vi "Main_flow_full_mqtt_with_power_calculation.vi"() -> ()   [LabVIEW 2022 SP3]
uses:
  D:/UOM/EE2044 - Electrical Measurements and Instrumentation/Project/Measurment Project/Quaxo_MQTT_LabVIEW-master/Controls/Connection_Return_Codes.ctl
  D:/UOM/EE2044 - Electrical Measurements and Instrumentation/Project/Measurment Project/Quaxo_MQTT_LabVIEW-master/Controls/QoS.ctl
  D:/UOM/EE2044 - Electrical Measurements and Instrumentation/Project/Measurment Project/Quaxo_MQTT_LabVIEW-master/Controls/Retain_Flag.ctl
  D:/UOM/EE2044 - Electrical Measurements and Instrumentation/Project/Measurment Project/Quaxo_MQTT_LabVIEW-master/Controls/DUP_Flag.ctl
  D:/UOM/EE2044 - Electrical Measurements and Instrumentation/Project/Measurment Project/Quaxo_MQTT_LabVIEW-master/Controls/Connect_Flags.ctl
  D:/UOM/EE2044 - Electrical Measurements and Instrumentation/Project/Measurment Project/Quaxo_MQTT_LabVIEW-master/Controls/User_Info.ctl
  <vilib>/DAQmx/write.llb/DAQmx Write (Digital Bool 1Line 1Point).vi
  <vilib>/DAQmx/read.llb/DAQmx Read (Digital Bool 1Line 1Point).vi
  <vilib>/DAQmx/create/channels.llb/DAQmx Create Channel (DO-Digital Output).vi
  <vilib>/DAQmx/create/channels.llb/DAQmx Create Channel (DI-Digital Input).vi
  <vilib>/DAQmx/miscellaneous.llb/DAQmx Fill In Error Info.vi
  <vilib>/DAQmx/create/channels.llb/DAQmx Create Channel (AI-Voltage-Basic).vi
  <vilib>/DAQmx/read.llb/DAQmx Read (Analog 1D DBL NChan 1Samp).vi
  D:/UOM/EE2044 - Electrical Measurements and Instrumentation/Project/Measurment Project/Quaxo_MQTT_LabVIEW-master/MQTT_Functions.lvlib
panel:
  out "Current":dbl caption="Current (A)"
  out "Energy":dbl caption="Energy( Whr)"
  in  "clock stop":bool
  out "Time":string
  out "Servo Angle":dbl(knob) scale=0.0..150.0
  in  "stop (F)":bool
  out "PWM Wave":dynamicdata(graph) caption="Square"
  in  "Frequency":dbl=50.0
  in  "Offset":dbl=2.5
  in  "Amplitude":dbl=2.5
  in  "MQTT Broker":cluster{"address (IP)":string, "port":u16}={"address (IP)"="broker.mqttdashboard.com", "port"=1883}
  out "Counter":dbl
  out "OUT COUNT":dbl
  out "IN COUNT":dbl
  in  "Mode":dbl
  in  "Relay 2":tag
  in  "Relay 1":tag
  in  "UP DOWN 2":tag
  in  "UP DOWN 1":tag
  in  "Buzzer":tag
  in  "Door IR 1 & 2 & LDR & Current":tag
  out "LDR Value":dbl(knob) scale=0.0..10.0
  in  "Trigger Period(sec)":dbl
  out "?":bool
  out "?":bool
  out "?":bool
  in  "mqtt stop":bool
  in  "Publish Meta":cluster{"QoS":T1, "Retain":T2, "DUP":T3}
  out "Connection Status":T4=enum."Connection refused: not authorized"
  in  "Client ID":string="NodeE-12345"
  out "main loop executed":dbl
  out "Current Time":dbl
  in  "stop":bool
  # "Channel Configure"
  # "MQTT Configure"
  # "MQTT publish interval\nset channels\nset check mode trigger period"
  # "Dev1/ai4:7"
  # "Dev1/port0/line2"
  # "Dev1/port0/line0"
  # "Dev1/port0/line1"
  # "Dev1/port0/line3"
  # "Dev1/port0/line4"
  # "Dev1/port0/line4"
  # "Servo Motor Controller"
  # "Counter Status"
  # "Light Mode"
  # "Low"
  # "Medium"
  # "High"
  # "This Indicate the status of light mode in the room"
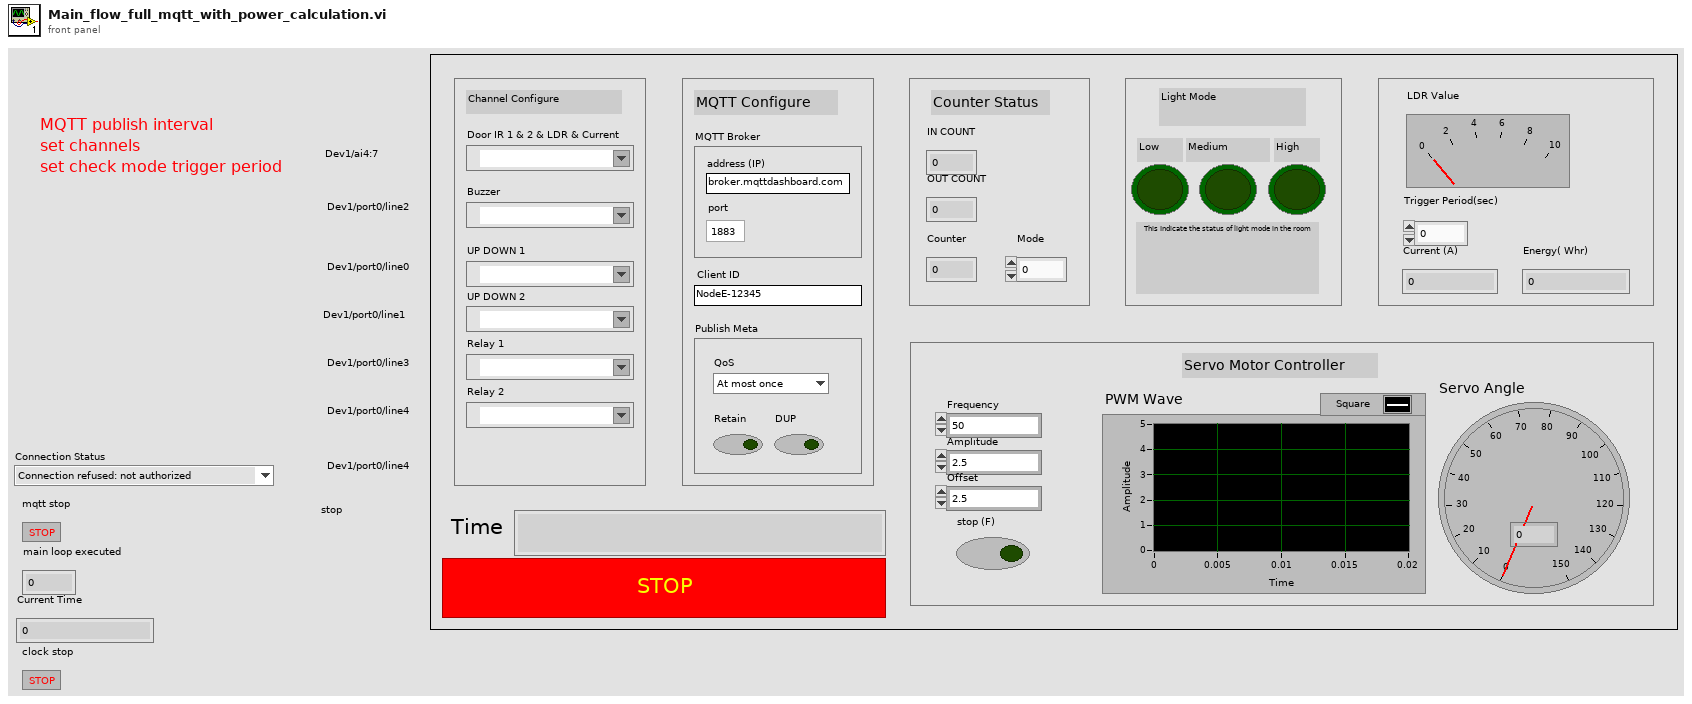
[diagram p1: front panel]
types:
  T1 = typedef "MQTT_Functions.lvlib/QoS.ctl" = enum8{"At most once", "At least once", "Exactly once", "Reserved"}
  T2 = typedef "MQTT_Functions.lvlib/Retain_Flag.ctl" = bool
  T3 = typedef "MQTT_Functions.lvlib/DUP_Flag.ctl" = bool
  T4 = typedef "MQTT_Functions.lvlib/Connection_Return_Codes.ctl" = enum16{"Connection accepted", "Connection refused: unacceptable protocol version", "Connection refused: identifier rejected", "Connection refused: Server unavailable", "Connection refused: bad user name or password", "Connection refused: not authorized"}
  T5 = typedef "MQTT_Functions.lvlib/User_Info.ctl" = cluster{"User Name":string, "Password":string}
  T6 = typedef "MQTT_Functions.lvlib/Connect_Flags.ctl" = cluster{"user name":bool, "password":bool, "will retain":bool, "will flag":bool, "clean session":bool, "reserved":bool, "will QoS":T1}
  T7 = cluster{"QoS":T1, "DUP":T3, "Retain":T2, "Keep Alive (sec)":u16}
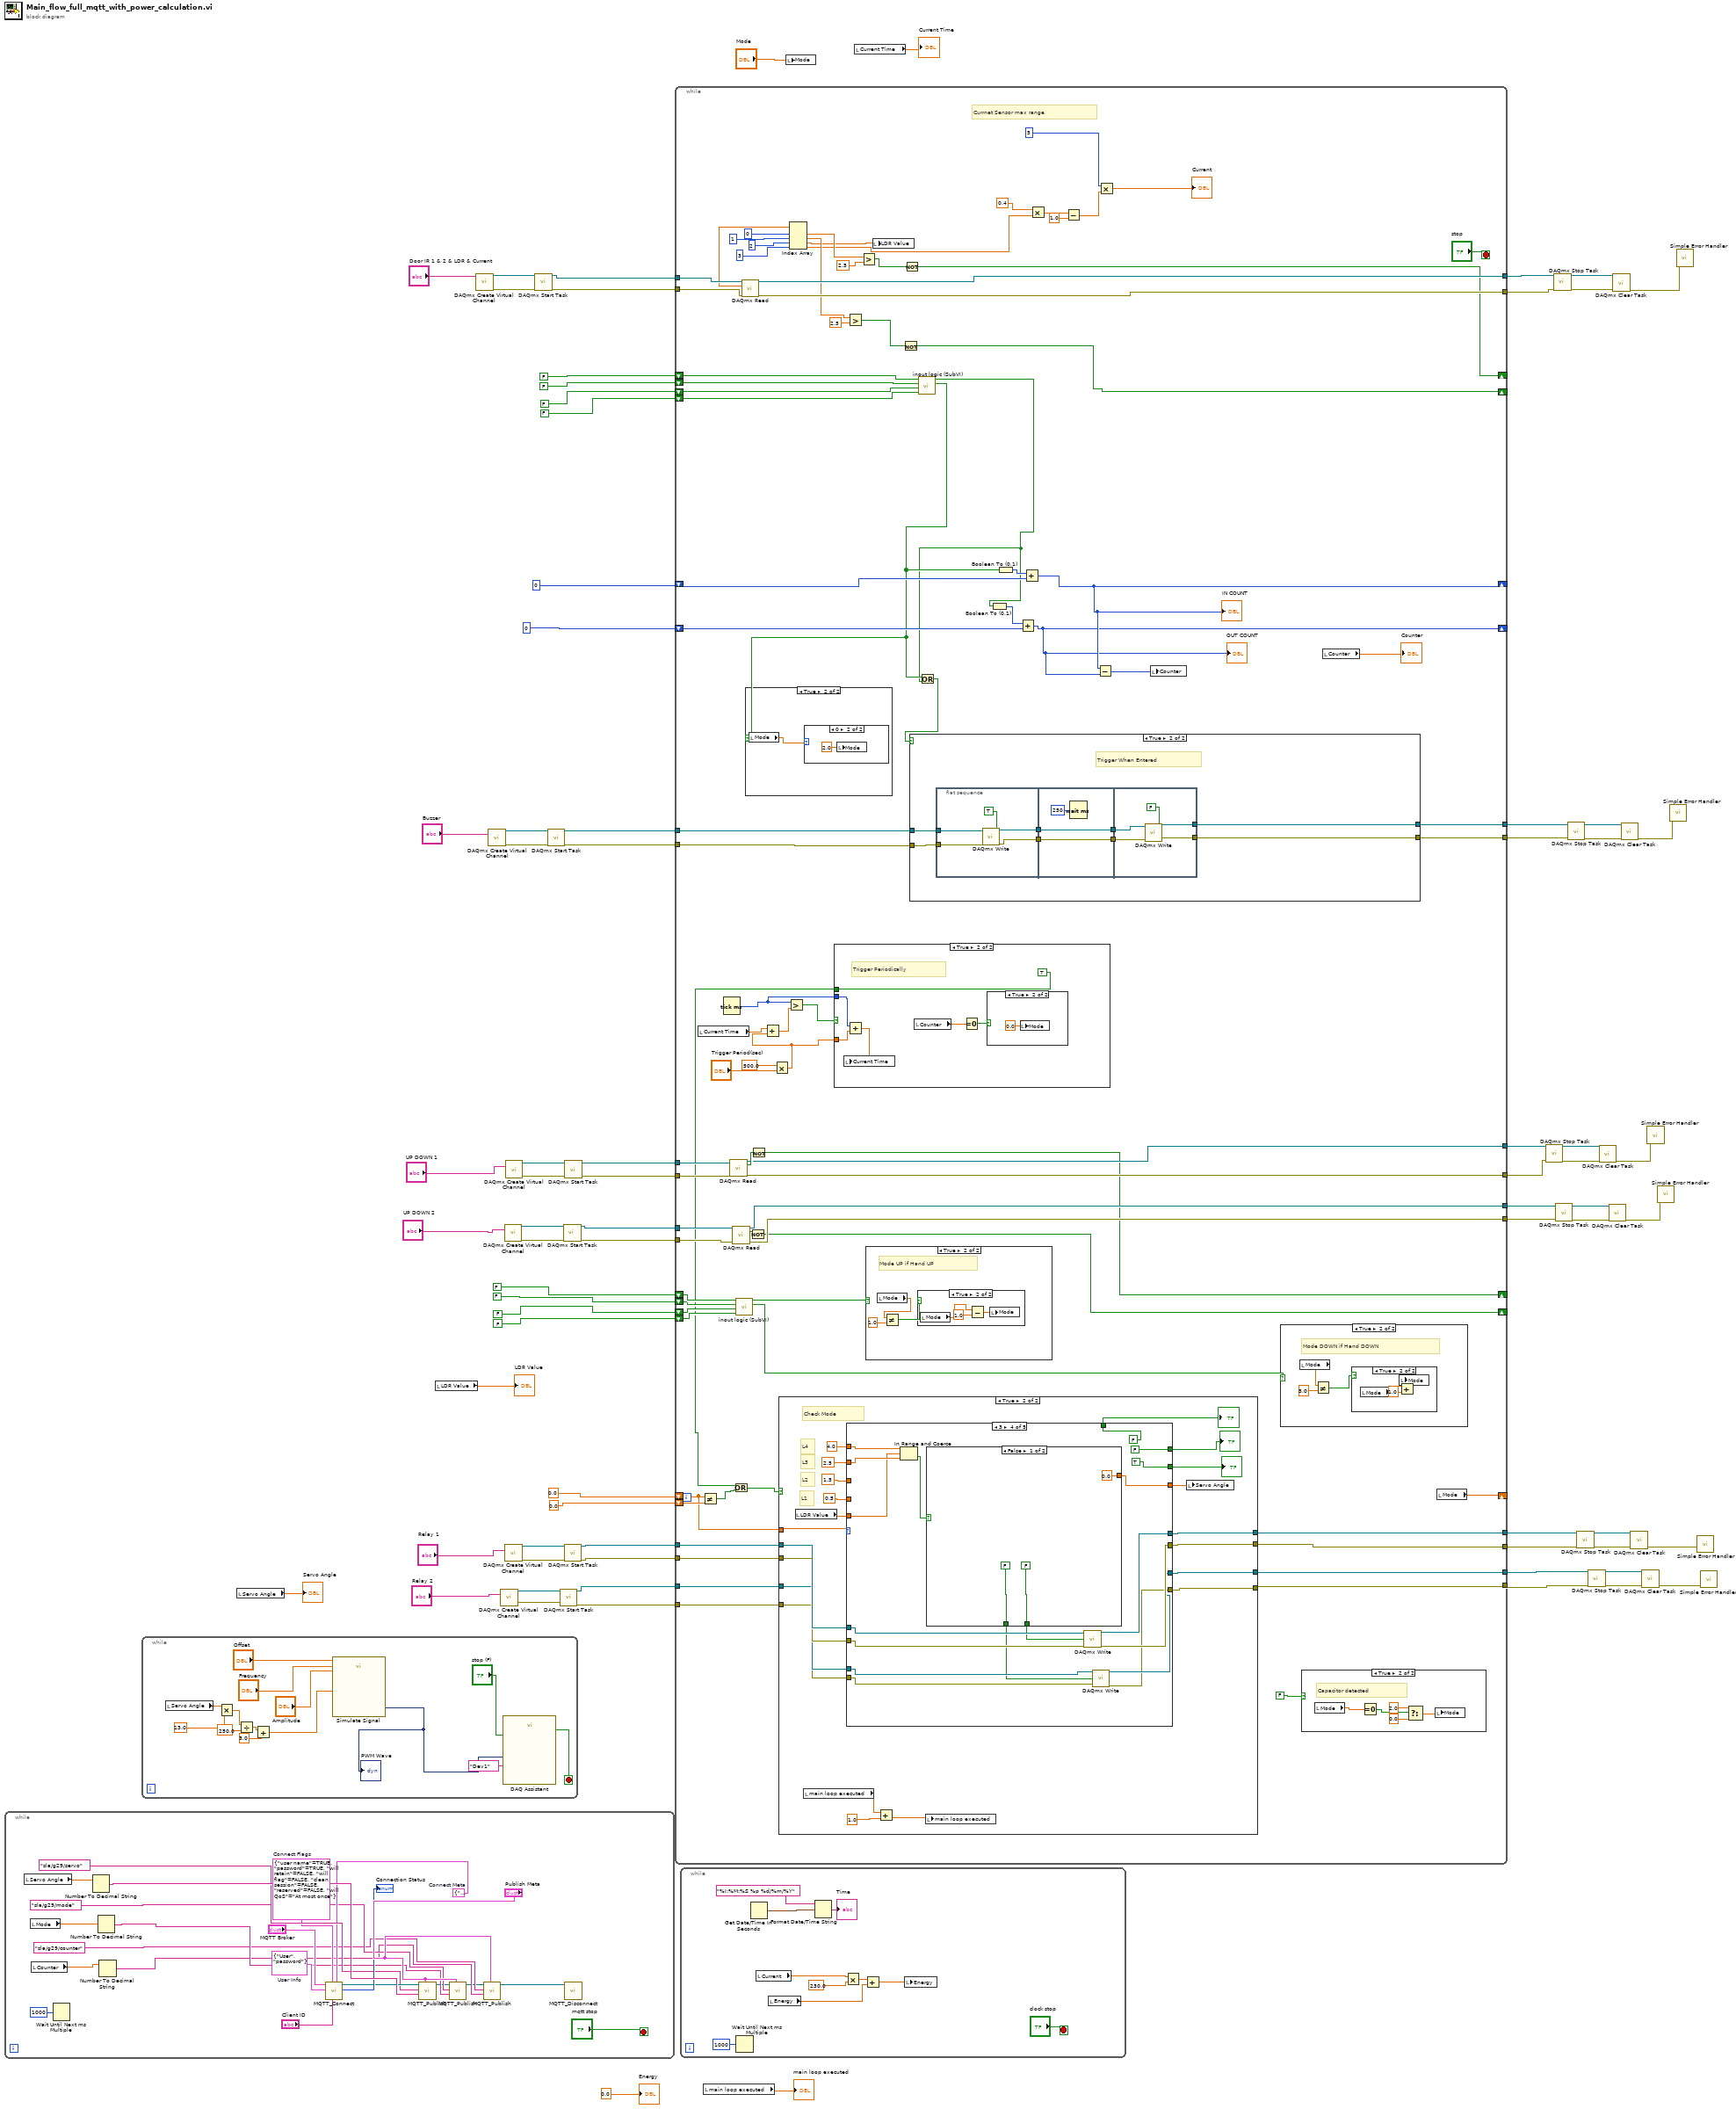
[diagram p0: block diagram]
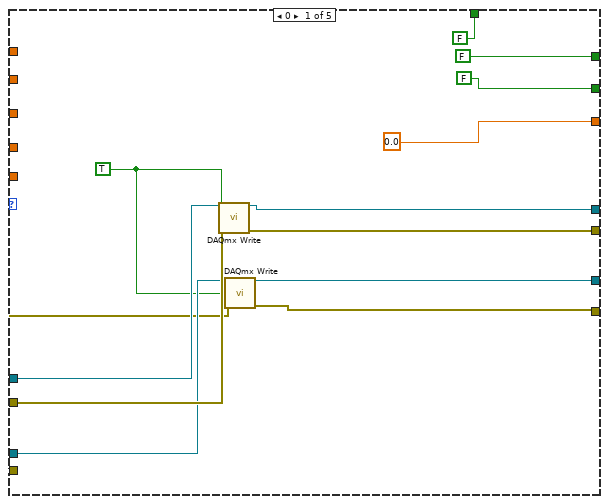
[diagram p5: hidden frame]
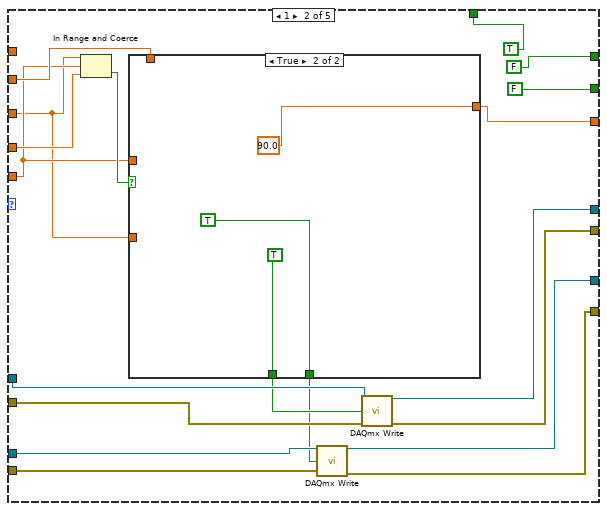
[diagram p6: hidden frame]
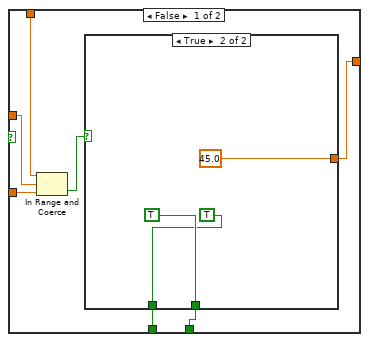
[diagram p7: hidden frame]
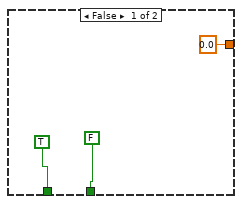
[diagram p8: hidden frame]
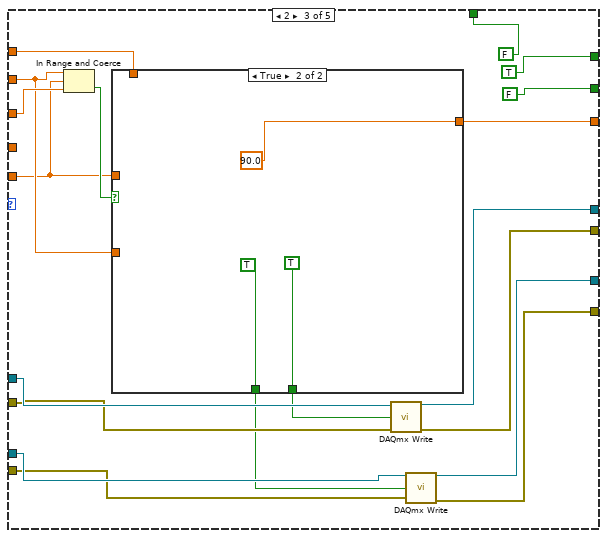
[diagram p9: hidden frame]
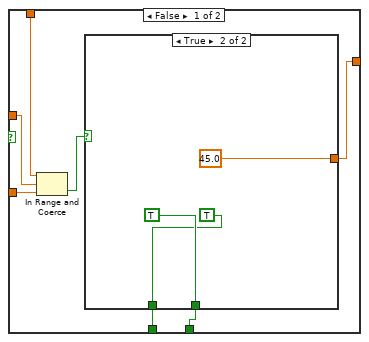
[diagram p10: hidden frame]
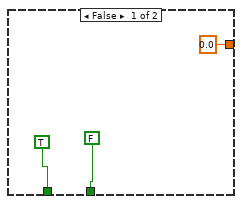
[diagram p11: hidden frame]
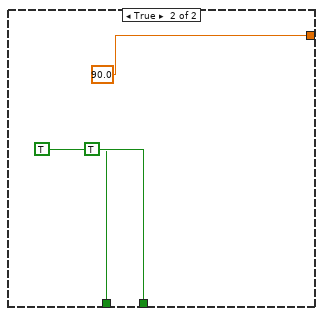
[diagram p12: hidden frame]
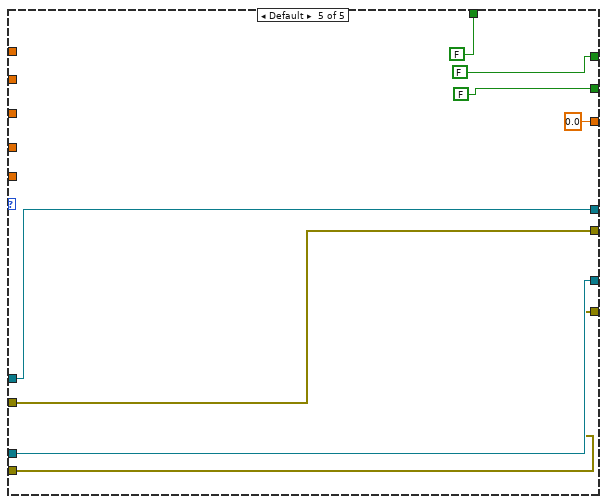
[diagram p13: hidden frame]
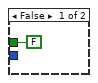
[diagram p18: hidden frame]
diagram:
  n1 = while {
    stop <- "mqtt stop" stop-if-true
    w86 = T5 {"User Name"="User", "Password"="password"}  # User Info
    w87 = T6 {"user name"=TRUE, "password"=TRUE, "will retain"=FALSE, "will flag"=FALSE, "clean session"=FALSE, "reserved"=FALSE, "will QoS"=enum."At most once"}  # Connect Flags
    w88 = T7 {"QoS"=enum."At most once", "DUP"=FALSE, "Retain"=FALSE, "Keep Alive (sec)"=60}  # Connect Meta
    n2 = local read "Servo Angle"() -> (w97:dbl)
    n3 = local read "Mode"() -> (w99:dbl)
    n4 = local read "Counter"() -> (w98:dbl)
    n5 = Wait Until Next ms Multiple(millisecond multiple=u32 1000) -> ()  [unwired: 1 out]
    n6 = Number To Decimal String(number=w97) -> (decimal integer string=w96:string)  [unwired: 1 in]
    n7 = Number To Decimal String(number=w99) -> (decimal integer string=w85:string)  [unwired: 1 in]
    n8 = Number To Decimal String(number=w98) -> (decimal integer string=w83:string)  [unwired: 1 in]
    n9 = call "MQTT_Connect.vi"("Connect Meta"=w88, "Client ID"="Client ID", "Connect Flags"=w87, "User Info"=w86, "MQTT Broker"="MQTT Broker") -> ("Connection Status"=→"Connection Status":T4, "connection ID out"=w93:refnum<k5>)  [unwired: 4 in, 1 out]
    n10 = call "MQTT_Publish.vi"("Publish Meta"="Publish Meta", "Message to be published"=w96, "Topic"="sla/g29/servo", "connection ID"=w93) -> ("connection ID out"=w80:refnum<k5>)  [unwired: 6 in, 1 out]
    n11 = call "MQTT_Publish.vi"("Publish Meta"="Publish Meta", "Message to be published"=w85, "Topic"="sla/g29/mode", "connection ID"=w80) -> ("connection ID out"=w79:refnum<k5>)  [unwired: 6 in, 1 out]
    n12 = call "MQTT_Publish.vi"("Publish Meta"="Publish Meta", "Message to be published"=w83, "Topic"="sla/g29/counter", "connection ID"=w79) -> ("connection ID out"=w91:refnum<k5>)  [unwired: 6 in, 1 out]
    n13 = call "MQTT_Disconnect.vi"("connection ID"=w91) -> ()  [unwired: 10 in, 1 out]
  }
  n14 = while {
    stop <- w113 stop-if-true
    n15 = local read "Servo Angle"() -> (w101:dbl)
    n16 = Multiply(x=w101, y=13.0) -> (x*y=w107:dbl)
    n17 = Divide(x=w107, y=250.0) -> (x/y=w106:dbl)
    n18 = Add(x=w106, y=3.0) -> (x+y=w102:dbl)
    n19 = call "Simulate Signal"("Offset"="Offset", "Duty Cycle (%)"=w102, "Frequency"="Frequency", "Amplitude"="Amplitude") -> ("Square"=w109:dynamicdata)  [unwired: 10 in, 1 out]
    "PWM Wave" <- w109
    n20 = call "DAQ Assistant"("data"=w109, "stop (F)"="stop (F)", "device name"=tag "Dev1") -> ("stopped"=w113:bool)  [unwired: 14 in, 2 out]
  }
  n21 = local read "Servo Angle"() -> (→"Servo Angle":dbl)
  n22 = local read "LDR Value"() -> (→"LDR Value":dbl)
  n23 = call-poly <vilib>:"DAQmx Create Virtual Channel.vi"("physical channels"="Door IR 1 & 2 & LDR & Current") -> ("task out"=w74:refnum<k21>, "error out"=w71:errorcluster)  [unwired: 13 in]
  n24 = call-poly <vilib>:"DAQmx Create Virtual Channel.vi"("lines"="Buzzer") -> ("task out"=w59:refnum<k21>, "error out"=w57:errorcluster)  [unwired: 13 in]
  n25 = call-poly <vilib>:"DAQmx Create Virtual Channel.vi"("lines"="Relay 2") -> ("task out"=w20:refnum<k21>, "error out"=w19:errorcluster)  [unwired: 13 in]
  n26 = call-poly <vilib>:"DAQmx Create Virtual Channel.vi"("lines"="UP DOWN 2") -> ("task out"=w48:refnum<k21>, "error out"=w46:errorcluster)  [unwired: 13 in]
  n27 = call-poly <vilib>:"DAQmx Create Virtual Channel.vi"("lines"="Relay 1") -> ("task out"=w23:refnum<k21>, "error out"=w22:errorcluster)  [unwired: 13 in]
  n28 = call-poly <vilib>:"DAQmx Create Virtual Channel.vi"("lines"="UP DOWN 1") -> ("task out"=w49:refnum<k21>, "error out"=w47:errorcluster)  [unwired: 13 in]
  n29 = call <vilib>:"DAQmx Start Task.vi"("task/channels in"=w74, "error in"=w71) -> ("task out"=w72:refnum<k21>, "error out"=w70:errorcluster)  [unwired: 12 in]
  n30 = call <vilib>:"DAQmx Start Task.vi"("task/channels in"=w59, "error in"=w57) -> ("task out"=w56:refnum<k21>, "error out"=w55:errorcluster)  [unwired: 12 in]
  n31 = call <vilib>:"DAQmx Start Task.vi"("task/channels in"=w20, "error in"=w19) -> ("task out"=w15:refnum<k21>, "error out"=w14:errorcluster)  [unwired: 12 in]
  n32 = call <vilib>:"DAQmx Start Task.vi"("task/channels in"=w48, "error in"=w46) -> ("task out"=w41:refnum<k21>, "error out"=w40:errorcluster)  [unwired: 12 in]
  n33 = call <vilib>:"DAQmx Start Task.vi"("task/channels in"=w23, "error in"=w22) -> ("task out"=w17:refnum<k21>, "error out"=w16:errorcluster)  [unwired: 12 in]
  n34 = call <vilib>:"DAQmx Start Task.vi"("task/channels in"=w49, "error in"=w47) -> ("task out"=w43:refnum<k21>, "error out"=w42:errorcluster)  [unwired: 12 in]
  n35 = while {
    shift-right: [w191] -> _
    shift-left: 0.0 ("Mode") -> [w189]
    shift-left: 0.0 ("Mode") -> [w190]
    tunnel: w72 -> [w186]
    tunnel: w70 -> [w185]
    tunnel: [w184] -> w69
    tunnel: [w183] -> w68
    shift-right: [w174] -> _
    shift-left: FALSE -> [w182]
    shift-left: FALSE -> [w181]
    shift-right: [w177] -> _
    shift-left: FALSE -> [w180]
    shift-left: FALSE -> [w151]
    shift-right: [w176] -> _
    shift-left: 0 -> [w179]
    shift-right: [w175] -> _
    shift-left: 0 -> [w178]
    tunnel: w56 -> [w171]
    tunnel: w55 -> [w170]
    tunnel: [w169] -> w51
    tunnel: [w168] -> w50
    shift-right: [w157] -> _
    shift-left: FALSE -> [w155]
    shift-right: [w156] -> _
    shift-left: FALSE -> [w153]
    shift-left: FALSE -> [w154]
    shift-left: FALSE -> [w152]
    tunnel: w43 -> [w165]
    tunnel: w42 -> [w164]
    tunnel: w41 -> [w163]
    tunnel: w40 -> [w162]
    tunnel: [w161] -> w33
    tunnel: [w160] -> w32
    tunnel: [w159] -> w31
    tunnel: [w158] -> w30
    tunnel: w17 -> [w133]
    tunnel: w16 -> [w132]
    tunnel: w15 -> [w131]
    tunnel: w14 -> [w130]
    tunnel: [w129] -> w7
    tunnel: [w128] -> w6
    tunnel: [w127] -> w5
    tunnel: [w126] -> w4
    stop <- "stop" stop-if-true
    # "Currnet Sensor max range"
    n36 = local read "Current Time"() -> (w198:dbl)
    n37 = Not Equal?(x=w189, y=w190) -> (x != y?=w125:bool)
    n38 = Tick Count (ms)() -> (millisecond timer value=w196:u32)
    n39 = call-poly <vilib>:"DAQmx Read.vi"("task/channels in"=w165, "error in"=w164) -> ("task out"=w161:refnum<k21>, "data"=w167:bool, "error out"=w160:errorcluster)  [unwired: 11 in]
    n40 = call-poly <vilib>:"DAQmx Read.vi"("task/channels in"=w163, "error in"=w162) -> ("task out"=w159:refnum<k21>, "data"=w166:bool, "error out"=w158:errorcluster)  [unwired: 11 in]
    n41 = call "inout logic (SubVI).vi"("Sensor 2 (T-2)"=w152, "Sensor 2 (T-1)"=w153, "Sensor 1 (T-2)"=w154, "Sensor 1 (T-1)"=w155) -> ("IN"=w150:bool, "OUT"=w149:bool)  [unwired: 6 in]
    n42 = call-poly <vilib>:"DAQmx Read.vi"("task/channels in"=w186, "error in"=w185) -> ("task out"=w184:refnum<k21>, "data"=w143:dbl[], "error out"=w183:errorcluster)  [unwired: 11 in]
    n43 = Not(x=w166) -> (.not. x?=w156:bool)
    n44 = Not(x=w167) -> (.not. x?=w157:bool)
    n45 = Multiply(x=500.0, y="Trigger Period(sec)") -> (x*y=w192:dbl)
    n46 = Add(x=w198, y=w192) -> (x+y=w195:dbl)
    n47 = Greater?(x=w196, y=w195) -> (0:w197:bool)
    n48 = Index Array(array=w143, index #1=0 ("index"), index #2=1 ("index"), index #3=2 ("index"), index #4=3 ("index")) -> (element #1=w142:dbl, element #2=w139:dbl, element #3=w134:dbl, element #4=w115:dbl)
    n49 = case shown="True" w197 {
      tunnel: w196 -> [_ w359]
      tunnel: w192 -> [_ w358]
      tunnel: [FALSE ("Check") TRUE ("Check")] -> w123
      frame False {
      }
      frame True {
        # "Trigger Periodically"
        n50 = Add(x=w359, y=w358) -> (x+y=w360:dbl)
        n51 = local write "Current Time"(w360) -> ()
        n52 = local read "Counter"() -> (w357:dbl)
        n53 = Equal To 0?(x=w357) -> (x = 0?=w356:bool)
        n54 = case shown="True" w356 {
          frame False {
          }
          frame True {
            n55 = local write "Mode"(0.0 ("Mode")) -> ()
          }
        }
      }
    }
    n56 = Or(x=w123, y=w125) -> (x .or. y?=w124:bool)
    n57 = case shown="True" w124 {
      tunnel: w189 -> [_ w226]
      tunnel: w133 -> [w205 w225]
      tunnel: w132 -> [w204 w224]
      tunnel: w131 -> [w203 w223]
      tunnel: w130 -> [w202 w222]
      tunnel: [w205 w221] -> w129
      tunnel: [w204 w220] -> w128
      tunnel: [w203 w219] -> w127
      tunnel: [w202 w218] -> w126
      frame False {
      }
      frame True {
        # "L4"
        # "L1"
        # "L3"
        # "L2"
        # "Check Mode"
        n58 = local read "LDR Value"() -> (w216:dbl)
        n59 = local read "main loop executed"() -> (w211:dbl)
        n60 = case shown="3" w226 {
          tunnel: w225 -> [w239 w258 w293 w327 w341]
          tunnel: w224 -> [w238 w256 w292 w326 w340]
          tunnel: w223 -> [w237 w254 w291 w325 w339]
          tunnel: w222 -> [w236 w252 w290 w324 w338]
          tunnel: [w235 w257 w289 w323 w341] -> w221
          tunnel: [w234 w255 w288 w322 w340] -> w220
          tunnel: [w233 w253 w287 w321 w339] -> w219
          tunnel: [w232 w251 w286 w320 w338] -> w218
          tunnel: 1.5 -> [_ w246 w285 _ _]
          tunnel: 0.5 -> [_ w249 _ _ _]
          tunnel: w216 -> [_ w247 w278 w316 _]
          tunnel: 2.5 -> [_ w248 w279 w317 _]
          tunnel: 4.0 -> [_ _ w280 w318 _]
          tunnel: [0.0 ("Servo Angle") w243 w283 w315 0.0 ("A")] -> w212
          tunnel: [FALSE TRUE FALSE FALSE FALSE] -> w208
          tunnel: [FALSE FALSE TRUE FALSE FALSE] -> w207
          tunnel: [FALSE FALSE FALSE TRUE FALSE] -> w206
          frame 0 {
            w231 = TRUE ("data")
            n61 = call-poly <vilib>:"DAQmx Write.vi"("task/channels in"=w239, "data"=w231, "error in"=w238) -> ("task out"=w235:refnum<k21>, "error out"=w234:errorcluster)  [unwired: 10 in, 1 out]
            n62 = call-poly <vilib>:"DAQmx Write.vi"("task/channels in"=w237, "data"=w231, "error in"=w236) -> ("task out"=w233:refnum<k21>, "error out"=w232:errorcluster)  [unwired: 10 in, 1 out]
          }
          frame 1 {
            n63 = In Range and Coerce(upper limit=w246, x=w247, lower limit=w249) -> (In Range?=w250:bool)  [unwired: 1 out]
            n64 = case shown="True" w250 {
              tunnel: [w261 90.0] -> w243
              tunnel: [w260 TRUE] -> w244
              tunnel: [w259 TRUE] -> w245
              tunnel: w248 -> [w265 _]
              tunnel: w246 -> [w264 _]
              tunnel: w247 -> [w263 _]
              frame False {
                n65 = In Range and Coerce(upper limit=w265, x=w263, lower limit=w264) -> (In Range?=w262:bool)  [unwired: 1 out]
                n66 = case shown="True" w262 {
                  tunnel: [0.0 45.0] -> w261
                  tunnel: [FALSE TRUE] -> w260
                  tunnel: [TRUE TRUE] -> w259
                  frame False {
                  }
                  frame True {
                  }
                }
              }
              frame True {
              }
            }
            n67 = call-poly <vilib>:"DAQmx Write.vi"("task/channels in"=w254, "data"=w244, "error in"=w252) -> ("task out"=w253:refnum<k21>, "error out"=w251:errorcluster)  [unwired: 10 in, 1 out]
            n68 = call-poly <vilib>:"DAQmx Write.vi"("task/channels in"=w258, "data"=w245, "error in"=w256) -> ("task out"=w257:refnum<k21>, "error out"=w255:errorcluster)  [unwired: 10 in, 1 out]
          }
          frame 2 {
            n69 = In Range and Coerce(upper limit=w279, x=w278, lower limit=w285) -> (In Range?=w284:bool)  [unwired: 1 out]
            n70 = case shown="True" w284 {
              tunnel: [w296 90.0] -> w283
              tunnel: [w295 TRUE] -> w282
              tunnel: [w294 TRUE] -> w281
              tunnel: w280 -> [w300 _]
              tunnel: w279 -> [w299 _]
              tunnel: w278 -> [w298 _]
              frame False {
                n71 = In Range and Coerce(upper limit=w300, x=w298, lower limit=w299) -> (In Range?=w297:bool)  [unwired: 1 out]
                n72 = case shown="True" w297 {
                  tunnel: [0.0 45.0] -> w296
                  tunnel: [FALSE TRUE] -> w295
                  tunnel: [TRUE TRUE] -> w294
                  frame False {
                  }
                  frame True {
                  }
                }
              }
              frame True {
              }
            }
            n73 = call-poly <vilib>:"DAQmx Write.vi"("task/channels in"=w293, "data"=w282, "error in"=w292) -> ("task out"=w289:refnum<k21>, "error out"=w288:errorcluster)  [unwired: 10 in, 1 out]
            n74 = call-poly <vilib>:"DAQmx Write.vi"("task/channels in"=w291, "data"=w281, "error in"=w290) -> ("task out"=w287:refnum<k21>, "error out"=w286:errorcluster)  [unwired: 10 in, 1 out]
          }
          frame 3 {
            n75 = In Range and Coerce(upper limit=w318, x=w316, lower limit=w317) -> (In Range?=w319:bool)  [unwired: 1 out]
            n76 = case shown="False" w319 {
              tunnel: [0.0 90.0] -> w315
              tunnel: [FALSE TRUE] -> w314
              tunnel: [FALSE TRUE] -> w313
              frame False {
              }
              frame True {
              }
            }
            n77 = call-poly <vilib>:"DAQmx Write.vi"("task/channels in"=w327, "data"=w314, "error in"=w326) -> ("task out"=w323:refnum<k21>, "error out"=w322:errorcluster)  [unwired: 10 in, 1 out]
            n78 = call-poly <vilib>:"DAQmx Write.vi"("task/channels in"=w325, "data"=w313, "error in"=w324) -> ("task out"=w321:refnum<k21>, "error out"=w320:errorcluster)  [unwired: 10 in, 1 out]
          }
          frame Default {
          }
        }
        "?" <- w206
        "?" <- w207
        "?" <- w208
        n79 = Add(x=w211, y=1.0) -> (x+y=w209:dbl)
        n80 = local write "main loop executed"(w209) -> ()
        n81 = local write "Servo Angle"(w212) -> ()
      }
    }
    n82 = Greater?(x=w139, y=2.5) -> (0:w145:bool)
    n83 = Greater?(x=w142, y=2.5) -> (0:w147:bool)
    n84 = case shown="True" w149 {
      frame False {
      }
      frame True {
        # "Mode UP if Hand UP"
        n85 = local read "Mode"() -> (w344:dbl)
        n86 = Not Equal?(x=w344, y=1.0) -> (x != y?=w343:bool)
        n87 = case shown="True" w343 {
          frame False {
          }
          frame True {
            n88 = local read "Mode"() -> (w346:dbl)
            n89 = Subtract(x=w346, y=1.0) -> (x-y=w345:dbl)
            n90 = local write "Mode"(w345) -> ()
          }
        }
      }
    }
    n91 = local write "LDR Value"(w134) -> ()
    n92 = Not(x=w145) -> (.not. x?=w177:bool)
    n93 = Not(x=w147) -> (.not. x?=w174:bool)
    n94 = call "inout logic (SubVI).vi"("Sensor 2 (T-2)"=w151, "Sensor 2 (T-1)"=w180, "Sensor 1 (T-2)"=w181, "Sensor 1 (T-1)"=w182) -> ("IN"=w138:bool, "OUT"=w137:bool)  [unwired: 6 in]
    n95 = case shown="True" w138 {
      frame False {
      }
      frame True {
        n96 = local read "Mode"() -> (w200:dbl)
        n97 = case shown="0" w200 {
          frame Default {
          }
          frame 0 {
            n98 = local write "Mode"(2.0 ("Mode")) -> ()
          }
        }
      }
    }
    n99 = Or(x=w138, y=w137) -> (x .or. y?=w136:bool)
    n100 = case shown="True" w136 {
      tunnel: w171 -> [w362 w371]
      tunnel: w170 -> [w363 w370]
      tunnel: [w362 w365] -> w169
      tunnel: [w363 w364] -> w168
      frame False {
      }
      frame True {
        # "Trigger When Entered"
        n101 = flat-sequence {
          tunnel: w371 -> [w375]
          tunnel: w370 -> [w374]
          tunnel: [w373] -> w368
          tunnel: [w372] -> w366
          tunnel: [w378] -> w369
          tunnel: w368 -> [w378]
          tunnel: [w377] -> w367
          tunnel: w366 -> [w377]
          tunnel: w369 -> [w383]
          tunnel: w367 -> [w382]
          tunnel: [w381] -> w365
          tunnel: [w380] -> w364
          frame #0 {
            n102 = call-poly <vilib>:"DAQmx Write.vi"("task/channels in"=w375, "data"=TRUE, "error in"=w374) -> ("task out"=w373:refnum<k21>, "error out"=w372:errorcluster)  [unwired: 10 in, 1 out]
          }
          frame #1 {
            n103 = Wait (ms)(milliseconds to wait=u32 250) -> ()  [unwired: 1 out]
          }
          frame #2 {
            n104 = call-poly <vilib>:"DAQmx Write.vi"("task/channels in"=w383, "data"=FALSE, "error in"=w382) -> ("task out"=w381:refnum<k21>, "error out"=w380:errorcluster)  [unwired: 10 in, 1 out]
          }
        }
      }
    }
    n105 = Boolean To (0,1)(Boolean=w137) -> (0, 1=w187:i16)
    n106 = Boolean To (0,1)(Boolean=w138) -> (0, 1=w188:i16)
    n107 = Add(x=w187, y=w178) -> (x+y=w175:i32)
    "OUT COUNT" <- w175
    n108 = Add(x=w188, y=w179) -> (x+y=w176:i32)
    "IN COUNT" <- w176
    n109 = Multiply(x=0.4, y=w115) -> (x*y=w121:dbl)
    n110 = Subtract(x=w121, y=1.0) -> (x-y=w119:dbl)
    n111 = Subtract(x=w176, y=w175) -> (x-y=w173:i32)
    n112 = Multiply(x=5, y=w119) -> (x*y=→"Current":dbl)
    n113 = local write "Counter"(w173) -> ()
    n114 = case shown="True" w150 {
      frame False {
      }
      frame True {
        # "Mode DOWN if Hand DOWN"
        n115 = local read "Mode"() -> (w350:dbl)
        n116 = Not Equal?(x=w350, y=3.0) -> (x != y?=w348:bool)
        n117 = case shown="True" w348 {
          frame False {
          }
          frame True {
            n118 = local read "Mode"() -> (w353:dbl)
            n119 = Add(x=w353, y=1.0) -> (x+y=w351:dbl)
            n120 = local write "Mode"(w351) -> ()
          }
        }
      }
    }
    n121 = case shown="True" FALSE {
      frame False {
      }
      frame True {
        # "Capacitor detected"
        n122 = local read "Mode"() -> (w385:dbl)
        n123 = Equal To 0?(x=w385) -> (x = 0?=w386:bool)
        n124 = Select(t=2.0, s=w386, f=0.0) -> (s? t:f=w389:dbl)
        n125 = local write "Mode"(w389) -> ()
      }
    }
    n126 = local read "Counter"() -> (→"Counter":dbl)
    n127 = local read "Mode"() -> (w191:dbl)
  }
  n128 = while {
    stop <- "clock stop" stop-if-true
    n129 = Wait Until Next ms Multiple(millisecond multiple=u32 1000) -> ()  [unwired: 1 out]
    n130 = Get Date/Time In Seconds() -> (seconds since 1Jan1904=w399:timestamp)
    n131 = local read "Current"() -> (w392:dbl)
    n132 = local read "Energy"() -> (w391:dbl)
    n133 = Format Date/Time String(time format string (%c)="%I:%M:%S %p %d/%m/%Y", seconds (now)=w399) -> (date/time string=→"Time":string)  [unwired: 1 in]
    n134 = Multiply(x=w392, y=230.0) -> (x*y=w393:dbl)
    n135 = Add(x=w393, y=w391) -> (x+y=w390:dbl)
    n136 = local write "Energy"(w390) -> ()
  }
  n137 = local read "main loop executed"() -> (→"main loop executed":dbl)
  n138 = local write "Mode"("Mode") -> ()
  n139 = local read "Current Time"() -> (→"Current Time":dbl)
  n140 = call <vilib>:"DAQmx Stop Task.vi"("task/channels in"=w33, "error in"=w32) -> ("task out"=w39:refnum<k21>, "error out"=w37:errorcluster)  [unwired: 12 in]
  n141 = call <vilib>:"DAQmx Stop Task.vi"("task/channels in"=w69, "error in"=w68) -> ("task out"=w67:refnum<k21>, "error out"=w66:errorcluster)  [unwired: 12 in]
  n142 = call <vilib>:"DAQmx Stop Task.vi"("task/channels in"=w31, "error in"=w30) -> ("task out"=w36:refnum<k21>, "error out"=w34:errorcluster)  [unwired: 12 in]
  n143 = call <vilib>:"DAQmx Stop Task.vi"("task/channels in"=w51, "error in"=w50) -> ("task out"=w54:refnum<k21>, "error out"=w52:errorcluster)  [unwired: 12 in]
  n144 = call <vilib>:"DAQmx Stop Task.vi"("task/channels in"=w7, "error in"=w6) -> ("task out"=w13:refnum<k21>, "error out"=w11:errorcluster)  [unwired: 12 in]
  n145 = call <vilib>:"DAQmx Stop Task.vi"("task/channels in"=w5, "error in"=w4) -> ("task out"=w10:refnum<k21>, "error out"=w8:errorcluster)  [unwired: 12 in]
  n146 = call <vilib>:"DAQmx Clear Task.vi"("task in"=w39, "error in"=w37) -> ("error out"=w38:errorcluster)  [unwired: 13 in]
  n147 = call <vilib>:"DAQmx Clear Task.vi"("task in"=w36, "error in"=w34) -> ("error out"=w35:errorcluster)  [unwired: 13 in]
  n148 = call <vilib>:"DAQmx Clear Task.vi"("task in"=w67, "error in"=w66) -> ("error out"=w65:errorcluster)  [unwired: 13 in]
  n149 = call <vilib>:"DAQmx Clear Task.vi"("task in"=w54, "error in"=w52) -> ("error out"=w53:errorcluster)  [unwired: 13 in]
  n150 = call <vilib>:"DAQmx Clear Task.vi"("task in"=w13, "error in"=w11) -> ("error out"=w12:errorcluster)  [unwired: 13 in]
  n151 = call <vilib>:"DAQmx Clear Task.vi"("task in"=w10, "error in"=w8) -> ("error out"=w9:errorcluster)  [unwired: 13 in]
  n152 = call <vilib>:"Simple Error Handler.vi"("error in (no error)"=w38) -> ()  [unwired: 4 in, 5 out]
  n153 = call <vilib>:"Simple Error Handler.vi"("error in (no error)"=w35) -> ()  [unwired: 4 in, 5 out]
  n154 = call <vilib>:"Simple Error Handler.vi"("error in (no error)"=w53) -> ()  [unwired: 4 in, 5 out]
  n155 = call <vilib>:"Simple Error Handler.vi"("error in (no error)"=w65) -> ()  [unwired: 4 in, 5 out]
  n156 = call <vilib>:"Simple Error Handler.vi"("error in (no error)"=w12) -> ()  [unwired: 4 in, 5 out]
  n157 = call <vilib>:"Simple Error Handler.vi"("error in (no error)"=w9) -> ()  [unwired: 4 in, 5 out]
  "Energy" <- 0.0 ("Energy")
